vi "MS Operation IOP Ctrl.vi"(6 "PID Cluster":T3={"L1 to L4 PID Cluster"={"L1 PID Gains"={"Kp"=0.005, "Kd"=0.5, "Ki"=0.0005}, "L2 PID Gains"={"Kp"=0.01, "Kd"=1.0, "Ki"=0.005}, "L3 PID Gains"={"Kp"=0.05, "Kd"=1.0, "Ki"=0.0005}, "L4 PID Gains"={"Kp"=0.1, "Kd"=0.1, "Ki"=0.0005}}, "Stage PID Cluster"={"Stage Z PID"={"Kp"=0.0005, "Kd"=0.001, "Ki"=0.0}, "Stage Y PID"={"Kp"=0.0003, "Kd"=0.01, "Ki"=0.0}, "Stage X PID"={"Kp"=0.0003, "Kd"=0.01, "Ki"=0.0}}, "OCT Z PID Gains"={"Kp"=0.0003, "Kd"=0.0001, "Ki"=0.01}}, 8 "error in":errorcluster, 9 "Offset Home 2 RCM":dbl[](array[numeric])=[0.0, 0.0, 0.0, 0.0], 10 "Prev Posit Cluster":T2={"Prev L1 to L4 Posit"=[-0.5319, -0.035669172703475985, -2.0566170657346783, 0.9099264705882353], "Prev Stage Posit"=[6.002553885707208, 5.996566124542428, 5.995469940427586], "Prev OCT Z Posit"=-0.0}, 11 "FPGA VI Reference In":refnum<k20>) -> (0 "error out":errorcluster, 2 "Last Posit Cluster":T1={"Last L1 to L4 Posit"=[0.0, 0.0, 0.0, 0.0], "Last Stage Posit"=[6.0, 6.0, 6.0], "Last OCT Z Posit"=0.0}, 3 "FPGA VI Reference Out":refnum<k20>)   [LabVIEW 2016]
uses:
  Global Variables.vi
  <vilib>/Platform/TimedLoop/XDataNode/wakeup.ctl
  <vilib>/Platform/TimedLoop/XDataNode/XDNodeRunTimeDep.lvlib
  <vilib>/Platform/TimedLoop/XDataNode/nitl_modes.ctl
  <vilib>/Platform/TimedLoop/XDataNode/timing_clust.ctl
  <vilib>/platform/TimedLoop/XDataNode/XDataNode.xnode
  <vilib>/rvi/interface/nirviReadWriteControl/nirviReadWriteControl.xnode
  Library/KevinLibraryAll/labview/KevLib01.lvlib
  FPGA Bitfiles/PhantomControlPI_FPGATarget_QuadCtr2_E2412E44.lvbitx
  IRISS_FPGA_IO.vi
  <vilib>/Utility/error.llb/Error Cluster From Error Code.vi
  <vilib>/rvi/errors/niLvFpgaAdjustHostInterfaceError.vi
  <vilib>/Utility/file.llb/Write Delimited Spreadsheet (DBL).vi
  <vilib>/Utility/file.llb/Write Delimited Spreadsheet (string).vi
  NiFpgaLv.dll
panel:
  out "Period [ms]":i64=10
  out "Acc Button 4":bool
  out "Accurus Remote cmd":T4
  out "L1 to L4 Remote cmd":sgl[](array[numeric])
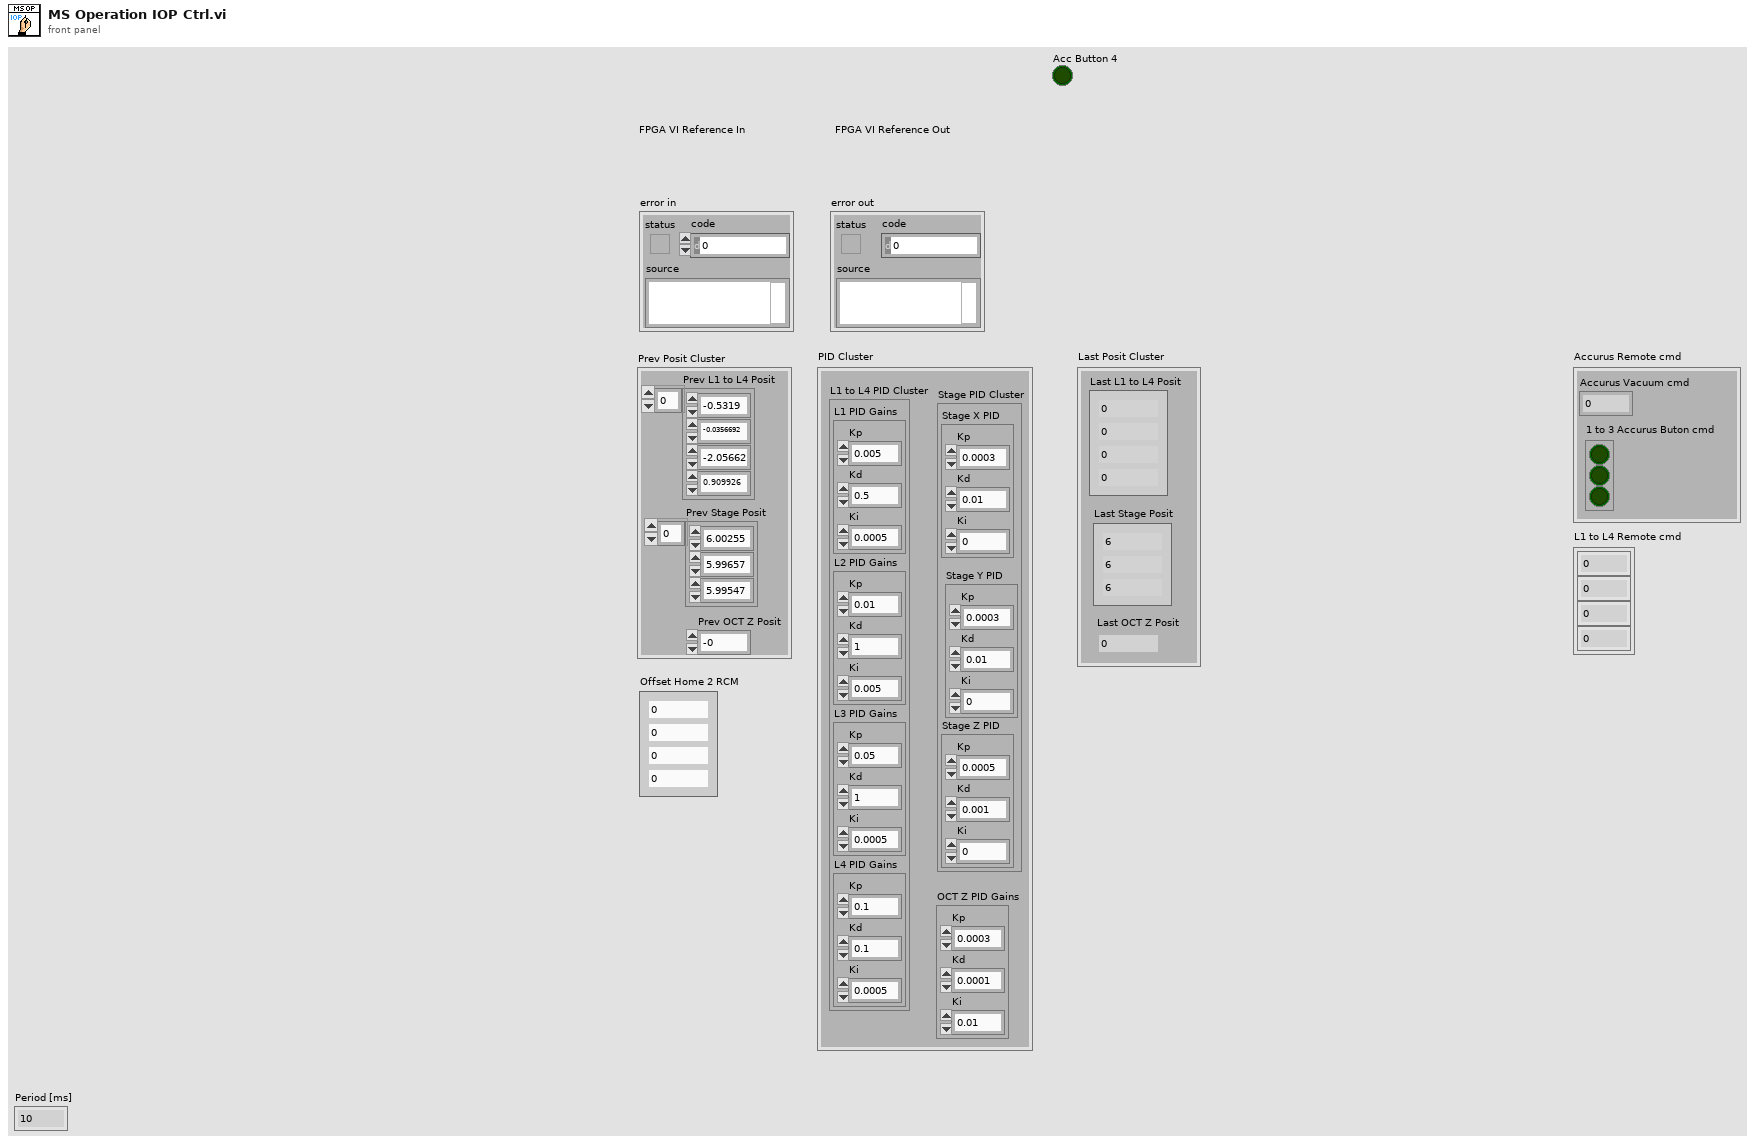
[diagram p1: front panel]
types:
  T1 = cluster{"Last L1 to L4 Posit":dbl[], "Last Stage Posit":dbl[], "Last OCT Z Posit":dbl}
  T2 = cluster{"Prev L1 to L4 Posit":dbl[], "Prev Stage Posit":dbl[], "Prev OCT Z Posit":dbl}
  T3 = cluster{"L1 to L4 PID Cluster":cluster{"L1 PID Gains":cluster{"Kp":dbl, "Kd":dbl, "Ki":dbl}, "L2 PID Gains":cluster{"Kp":dbl, "Kd":dbl, "Ki":dbl}, "L3 PID Gains":cluster{"Kp":dbl, "Kd":dbl, "Ki":dbl}, "L4 PID Gains":cluster{"Kp":dbl, "Kd":dbl, "Ki":dbl}}, "Stage PID Cluster":cluster{"Stage Z PID":cluster{"Kp":dbl, "Kd":dbl, "Ki":dbl}, "Stage Y PID":cluster{"Kp":dbl, "Kd":dbl, "Ki":dbl}, "Stage X PID":cluster{"Kp":dbl, "Kd":dbl, "Ki":dbl}}, "OCT Z PID Gains":cluster{"Kp":dbl, "Kd":dbl, "Ki":dbl}}
  T4 = cluster{"Accurus Vacuum cmd":sgl, "1 to 3 Accurus Buton cmd":bool[]}
  T5 = typedef "XDNodeRunTimeDep.lvlib/timing_clust.ctl" = cluster{"Expected End [f-1]":u64, "Actual End [f-1]":u64, "Finished Late? [f-1]":bool, "Expected End [i-1]":u64, "Actual End [i-1]":u64, "Finished Late? [i-1]":bool, "Expected Start [i]":u64, "Actual Start [i]":u64, "Expected Start [f]":u64, "Actual Start [f]":u64, "Source Name":string, "Structure Name":string, "Period":i64, "Deadline":i64, "Offset":i64, "Start":i64, "Priority":i32, "Timeout":i32, "Mode":T6, "Wakeup Reason":T7, "Error":errorcluster, "Source Type":string, "Secondary Source Type":string, "Global End Time":u64, "Global Start Time":u64, "Frame Duration":u64, "Iteration Duration":u64, "Assigned CPU":i32, "I/O Scan Engine Mode":u32}
  T6 = typedef "XDNodeRunTimeDep.lvlib/nitl_modes.ctl" = enum32{"No Change", "Process missed periods, maintain original phase", "Discard missed periods, maintain original phase", "Process missed periods, ignore original phase", "Discard missed periods, ignore original phase"}
  T7 = typedef "XDNodeRunTimeDep.lvlib/wakeup.ctl" = enum32{"Normal", "Aborted", "Asynchronous wakeup", "Timing source error", "Timed loop error", "Timeout"}
  T8 = cluster{"L1 PID Gains":cluster{"Kp":dbl, "Kd":dbl, "Ki":dbl}, "L2 PID Gains":cluster{"Kp":dbl, "Kd":dbl, "Ki":dbl}, "L3 PID Gains":cluster{"Kp":dbl, "Kd":dbl, "Ki":dbl}, "L4 PID Gains":cluster{"Kp":dbl, "Kd":dbl, "Ki":dbl}}
  T9 = cluster{"Stage Z PID":cluster{"Kp":dbl, "Kd":dbl, "Ki":dbl}, "Stage Y PID":cluster{"Kp":dbl, "Kd":dbl, "Ki":dbl}, "Stage X PID":cluster{"Kp":dbl, "Kd":dbl, "Ki":dbl}}
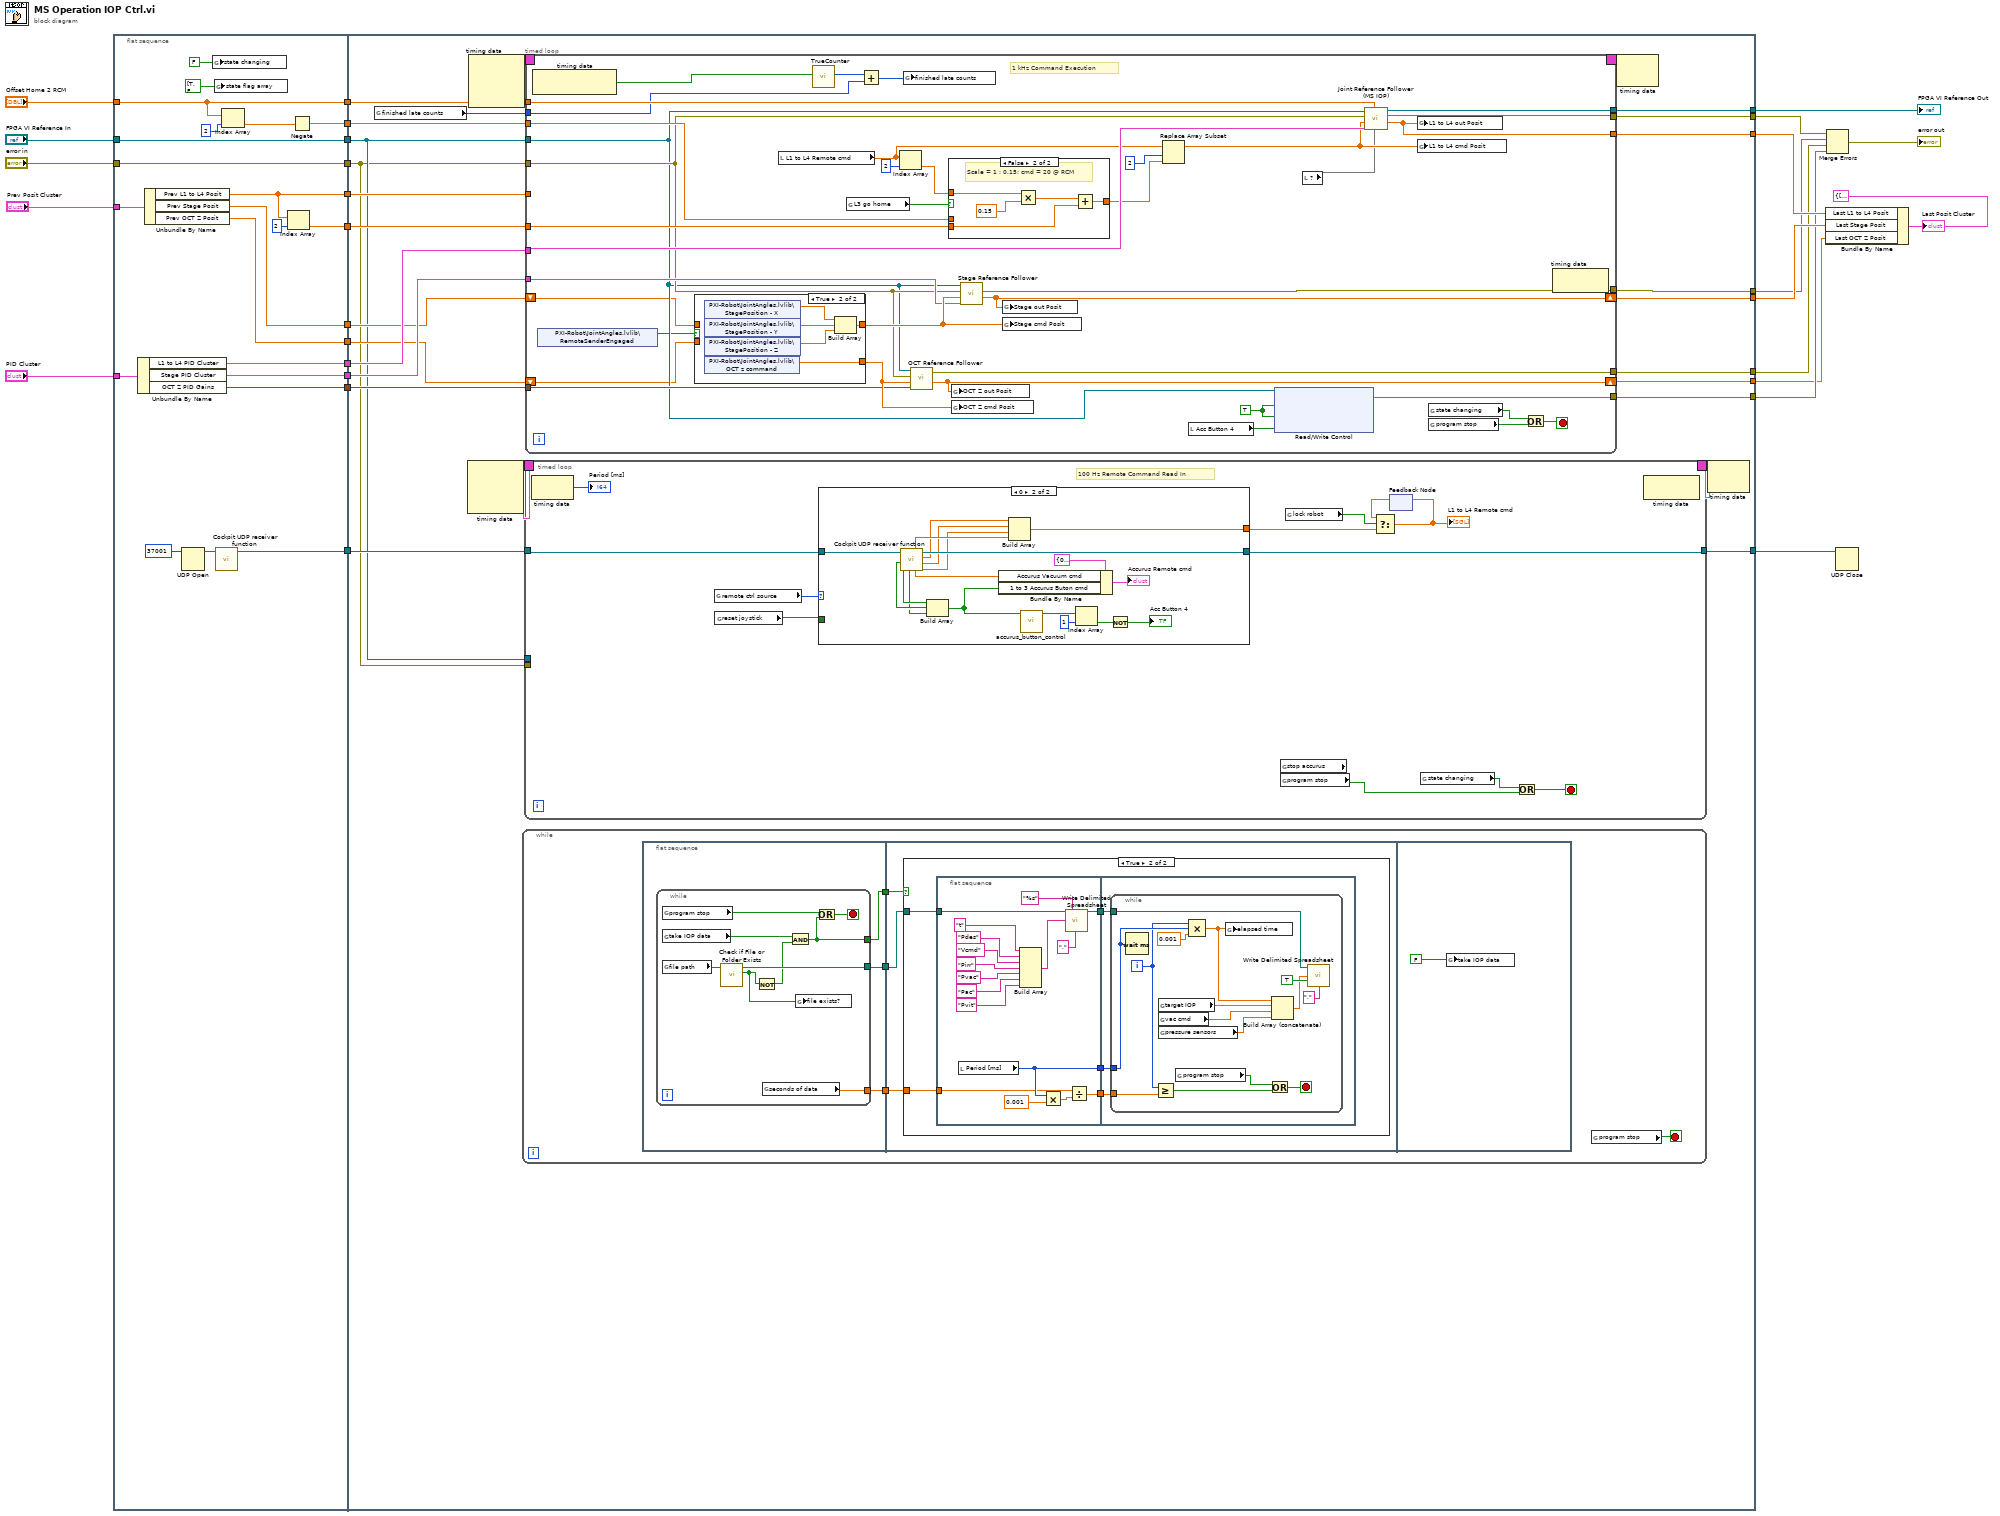
[diagram p0: block diagram]
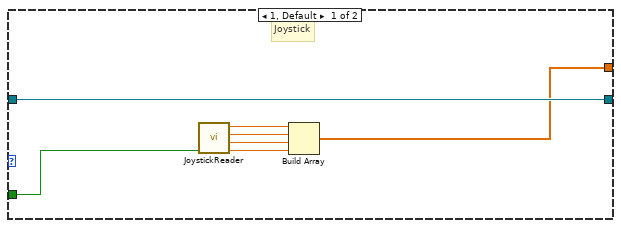
[diagram p3: hidden frame]
diagram:
  n1 = flat-sequence {
    tunnel: [w46] -> w29
    tunnel: [w45] -> w27
    tunnel: "FPGA VI Reference In" -> [w45]
    tunnel: [w44] -> w25
    tunnel: "error in" -> [w44]
    tunnel: [w37] -> w23
    tunnel: "Offset Home 2 RCM" -> [w37]
    tunnel: "Prev Posit Cluster" -> [w32]
    tunnel: [w42] -> w20
    tunnel: "PID Cluster" -> [w41]
    tunnel: [w40] -> w18
    tunnel: [w39] -> w17
    tunnel: [w35] -> w16
    tunnel: [w34] -> w4
    tunnel: [w33] -> w3
    tunnel: [w31] -> w2
    tunnel: [w30] -> w1
    tunnel: w29 -> [w72]
    tunnel: [w71] -> w28
    tunnel: w27 -> [w52]
    tunnel: w25 -> [w51]
    tunnel: w23 -> [w70]
    tunnel: w20 -> [w69]
    tunnel: w18 -> [w68]
    tunnel: w17 -> [w67]
    tunnel: w16 -> [w66]
    tunnel: [w65] -> w6
    tunnel: [w64] -> w12
    tunnel: [w63] -> w13
    tunnel: [w53] -> w10
    tunnel: [w54] -> w9
    tunnel: [w62] -> w7
    tunnel: [w61] -> w8
    tunnel: [w55] -> w5
    tunnel: w4 -> [w60]
    tunnel: w3 -> [w59]
    tunnel: w2 -> [w57]
    tunnel: w1 -> [w56]
    frame #0 {
      n2 = Unbundle By Name(w41) -> ("L1 to L4 PID Cluster"=w40:T8, "Stage PID Cluster"=w34:T9, "OCT Z PID Gains"=w33:cluster{"Kp":dbl, "Kd":dbl, "Ki":dbl})
      n3 = Unbundle By Name(w32) -> ("Prev L1 to L4 Posit"=w42:dbl[], "Prev Stage Posit"=w31:dbl[], "Prev OCT Z Posit"=w30:dbl)
      n4 = UDP Open(11:u16 37001 ("port")) -> (port=w48:refnum<k16>)  [unwired: 4 in, 2 out]
      n5 = global write "Global Variables.vi" "state changing"(FALSE ("state changing")) -> ()
      n6 = global write "Global Variables.vi" "state flag array"(bool[] [TRUE, FALSE, FALSE, FALSE, FALSE, FALSE, FALSE, FALSE, FALSE] ("state flag array")) -> ()
      n7 = call "Cockpit UDP receiver function.vi"("UDP connection ID"=w48) -> ("UDP connection ID out"=w46:refnum<k16>)  [unwired: 1 in, 9 out]
      n8 = Index Array(array=w37, index=2) -> (element=w36:dbl)
      n9 = Index Array(array=w42, index=2) -> (element=w39:dbl)
      n10 = Negate(x=w36) -> (-x=w35:dbl)
    }
    frame #1 {
      n11 = global read "Global Variables.vi" "finished late counts"() -> (w58:u16)
      n12 = node-c288() -> (w74:T5)  [unwired: 3 in]
      n13 = node-c288() -> (w76:T5)  [unwired: 3 in]
      n14 = while {
        stop <- w77 stop-if-true
        n15 = flat-sequence {
          tunnel: [w81] -> w80
          tunnel: [w83] -> w79
          tunnel: [w82] -> w78
          tunnel: w80 -> [w95]
          tunnel: w79 -> [w94]
          tunnel: w78 -> [w93]
          frame #0 {
            n16 = while {
              tunnel: [w91] -> w83
              tunnel: [w84] -> w82
              tunnel: [w89] -> w81
              stop <- w92 stop-if-true
              n17 = global read "Global Variables.vi" "program stop"() -> (w88:bool)
              n18 = global read "Global Variables.vi" "take IOP data"() -> (w87:bool)
              n19 = global read "Global Variables.vi" "file path"() -> (w86:path)
              n20 = call <vilib>:"Check if File or Folder Exists.vi"("path"=w86) -> ("file or folder exists?"=w85:bool, "dup path"=w91:path)  [unwired: 8 in, 1 out]
              n21 = Not(x=w85) -> (.not. x?=w90:bool)
              n22 = global read "Global Variables.vi" "seconds of data"() -> (w84:sgl)
              n23 = And(x=w87, y=w90) -> (x .and. y?=w89:bool)
              n24 = global write "Global Variables.vi" "file exists?"(w85) -> ()
              n25 = Or(x=w88, y=w89) -> (x .or. y?=w92:bool)
            }
          }
          frame #1 {
            n26 = case shown="True" w95 {
              tunnel: w94 -> [_ w100]
              tunnel: w93 -> [_ w97]
              frame False {
              }
              frame True {
                n27 = flat-sequence {
                  tunnel: w100 -> [w106]
                  tunnel: [w104] -> w99
                  tunnel: [w115] -> w98
                  tunnel: w97 -> [w114]
                  tunnel: [w112] -> w96
                  tunnel: w99 -> [w120]
                  tunnel: w98 -> [w119]
                  tunnel: w96 -> [w118]
                  frame #0 {
                    n28 = local read "Period [ms]"() -> (w115:i64)
                    n29 = Build Array("t" ("delimiter (\\t)"), "Pdes" ("delimiter (\\t)"), "Vcmd" ("delimiter (\\t)"), "Pirr" ("delimiter (\\t)"), "Pvac" ("delimiter (\\t)"), "Pac" ("delimiter (\\t)"), "Pvit" ("delimiter (\\t)")) -> (w103:string[])
                    n30 = Multiply(x=w115, y=0.001) -> (x*y=w113:dbl)
                    n31 = call-poly <vilib>:"Write Delimited Spreadsheet.vi"("file path (dialog if empty)"=w106, "format (%s)"="%s", "1D data"=w103, "delimiter (\\t)"="," ("delimiter (\\t)")) -> ("new file path (Not A Path if cancelled)"=w104:path)  [unwired: 10 in, 1 out]
                    n32 = Divide(x=w114, y=w113) -> (x/y=w112:dbl)
                  }
                  frame #1 {
                    n33 = while {
                      tunnel: w120 -> [w129]
                      tunnel: w119 -> [w133]
                      tunnel: w118 -> [w131]
                      i -> [w132]
                      stop <- w135 stop-if-true
                      n34 = Wait (ms)(milliseconds to wait=w133) -> ()  [unwired: 1 out]
                      n35 = Greater Or Equal?(x=w132, y=w131) -> (x >= y?=w130:bool)
                      n36 = global read "Global Variables.vi" "target IOP"() -> (w121:sgl)
                      n37 = global read "Global Variables.vi" "vac cmd"() -> (w124:sgl)
                      n38 = global read "Global Variables.vi" "pressure sensors"() -> (w123:sgl[])
                      n39 = global read "Global Variables.vi" "program stop"() -> (w125:bool)
                      n40 = Compound Arithmetic op=MULTIPLY(w132, w133, 0.001 ("y")) -> (w122:dbl)
                      n41 = global write "Global Variables.vi" "elapsed time"(w122) -> ()
                      n42 = Or(x=w125, y=w130) -> (x .or. y?=w135:bool)
                      n43 = Build Array (concatenate)(w122, w121, w124, w123) -> (w127:dbl[])
                      n44 = call-poly <vilib>:"Write Delimited Spreadsheet.vi"("file path (dialog if empty)"=w129, "1D data"=w127, "append to file? (new file:F)"=TRUE, "delimiter (\\t)"="," ("delimiter (\\t)")) -> ()  [unwired: 10 in, 2 out]
                    }
                  }
                }
              }
            }
          }
          frame #2 {
            n45 = global write "Global Variables.vi" "take IOP data"(FALSE) -> ()
          }
        }
        n46 = global read "Global Variables.vi" "program stop"() -> (w77:bool)
      }
      n47 = timed-loop {
        timing: w74 -> [_]
        timing-out: [_] -> w73
        tunnel: w72 -> [w146]
        tunnel: [w145] -> w71
        tunnel: w52 -> [_]
        tunnel: w51 -> [_]
        stop <- w148 stop-if-true
        # "100 Hz Remote Command Read In"
        n48 = node-c288() -> (→"Period [ms]":i64)  [unwired: 1 in]
        n49 = global read "Global Variables.vi" "remote ctrl source"() -> (w144:u16)
        n50 = global read "Global Variables.vi" "reset joystick"() -> (w143:bool)
        n51 = case shown="0" w144 {
          tunnel: [w154 w173] -> w145
          tunnel: w146 -> [w154 w163]
          tunnel: w143 -> [w155 _]
          tunnel: [w149 w162] -> w139
          frame 1, Default {
            # "Joystick"
            n52 = call "JoystickReader.vi"("Reset"=w155) -> ("L4 [deg]"=w150:sgl, "L3 [0~100]"=w151:sgl, "L2 [deg]"=w152:sgl, "L1 [deg]"=w153:sgl)  [unwired: 7 in]
            n53 = Build Array(w153, w152, w151, w150) -> (w149:sgl[])
          }
          frame 0 {
            n54 = call "Cockpit UDP receiver function.vi"("UDP connection ID"=w163) -> ("L3"=w170:sgl, "L2"=w169:sgl, "L1"=w171:sgl, "UDP connection ID out"=w173:refnum<k16>, "down_pedal"=w161:sgl, "L4"=w172:sgl, "right_pedal"=w164:bool, "left_pedal"=w166:bool, "up_pedal"=w165:bool)  [unwired: 1 in, 1 out]
            n55 = Build Array(w166, w165, w164) -> (w156:bool[])
            n56 = Bundle By Name(cluster=T4 {"Accurus Vacuum cmd"=0.0, "1 to 3 Accurus Buton cmd"=[FALSE, FALSE, FALSE]} ("Accurus Cockpit cmd 2"), "Accurus Vacuum cmd"=w161, "1 to 3 Accurus Buton cmd"=w156) -> (→"Accurus Remote cmd":T4)
            n57 = Build Array(w171, w169, w170, w172) -> (w162:sgl[])
            n58 = call "accurus_button_control.vi"("Array in"=w156) -> ("Array out"=w159:bool[])  [unwired: 10 in]
            n59 = Index Array(array=w159, index=1) -> (element=w158:bool)
            n60 = Not(x=w158) -> (.not. x?=→"Acc Button 4":bool)
          }
        }
        n61 = global read "Global Variables.vi" "stop accurus"() -> ()  [unwired: 1 out]
        n62 = global read "Global Variables.vi" "program stop"() -> (w138:bool)
        n63 = global read "Global Variables.vi" "lock robot"() -> (w142:bool)
        n64 = feedback #1() -> (w141:sgl[])  [unwired: 1 in]
        n65 = Select(t=w141, s=w142, f=w139) -> (s? t:f=w140:sgl[])
        "L1 to L4 Remote cmd" <- w140
        n66 = feedback-in #1(w140) -> ()
        n67 = global read "Global Variables.vi" "state changing"() -> (w147:bool)
        n68 = Or(x=w147, y=w138) -> (x .or. y?=w148:bool)
        n69 = node-c288() -> ()  [unwired: 1 in, 1 out]
      }
      n70 = timed-loop {
        timing: w76 -> [_]
        timing-out: [_] -> w75
        tunnel: w52 -> [w189]
        tunnel: w51 -> [w190]
        tunnel: w70 -> [w211]
        tunnel: w69 -> [_]
        tunnel: w68 -> [w208]
        tunnel: w67 -> [w207]
        tunnel: w66 -> [w204]
        tunnel: [w203] -> w65
        tunnel: [w202] -> w64
        tunnel: [w201] -> w63
        tunnel: [w200] -> w62
        tunnel: [w199] -> w61
        tunnel: w60 -> [w196]
        tunnel: w59 -> [w195]
        tunnel: w58 -> [w191]
        shift-right: [w185] -> w54
        shift-left: w57 -> [w188]
        shift-right: [w186] -> w55
        shift-left: w56 -> [w187]
        tunnel: [w182] -> w53
        stop <- w216 stop-if-true
        w198 = TRUE ("Conn0/DIO15 Button 4")
        # "1 kHz Command Execution"
        n71 = node-c288() -> (w194:bool)  [unwired: 1 in]
        n72 = shared-variable "PXI-Robot\\JointAngles.lvlib\\RemoteSenderEngaged"() -> (w184:bool)  [unwired: 1 in, 1 out]
        n73 = case shown="True" w184 {
          tunnel: [w218 w223] -> w210
          tunnel: [w217 w219] -> w209
          tunnel: w188 -> [w218 _]
          tunnel: w187 -> [w217 _]
          frame False {
          }
          frame True {
            n74 = shared-variable "PXI-Robot\\JointAngles.lvlib\\StagePosition - X"() -> (w220:dbl)  [unwired: 1 in, 1 out]
            n75 = shared-variable "PXI-Robot\\JointAngles.lvlib\\StagePosition - Y"() -> (w221:dbl)  [unwired: 1 in, 1 out]
            n76 = shared-variable "PXI-Robot\\JointAngles.lvlib\\StagePosition - Z"() -> (w222:dbl)  [unwired: 1 in, 1 out]
            n77 = shared-variable "PXI-Robot\\JointAngles.lvlib\\OCT z command"() -> (w219:dbl)  [unwired: 1 in, 1 out]
            n78 = Build Array(w220, w221, w222) -> (w223:dbl[])
          }
        }
        n79 = local read "L1 to L4 Remote cmd"() -> (w183:sgl[])
        n80 = call "TrueCounter.vi"("True?"=w194) -> ("True Count"=w192:u16)  [unwired: 10 in]
        n81 = global read "Global Variables.vi" "L3 go home"() -> (w214:bool)
        n82 = Add(x=w192, y=w191) -> (x+y=w193:u16)
        n83 = Index Array(array=w183, index=2) -> (element=w212:sgl)
        n84 = global write "Global Variables.vi" "finished late counts"(w193) -> ()
        n85 = call "OCT Reference Follower.vi"("OCT Z PID Gains"=w195, "OCT  Z cmd Posit [mm]"=w209, "error in"=w190, "FPGA VI Reference In"=w189) -> ("OCT  Z out Posit [mm]"=w186:dbl, "error out"=w200:errorcluster)  [unwired: 5 in, 1 out]
        n86 = case shown="False" w214 {
          tunnel: [w224 w229] -> w205
          tunnel: w212 -> [_ w226]
          tunnel: w207 -> [_ w225]
          tunnel: w204 -> [w224 _]
          frame True {
            # "Go Home"
          }
          frame False {
            # "Scale = 1 : 0.15; cmd = 20 @ RCM"
            n87 = Multiply(x=w226, y=0.15) -> (x*y=w228:dbl)
            n88 = Add(x=w228, y=w225) -> (x+y=w229:dbl)
          }
        }
        n89 = global write "Global Variables.vi" "OCT Z out Posit"(w186) -> ()
        n90 = global write "Global Variables.vi" "OCT Z cmd Posit"(w209) -> ()
        n91 = call "Stage Reference Follower.vi"("Stage PID Cluster"=w196, "Stage cmd Posit [mm]"=w210, "error in"=w190, "FPGA VI Reference In"=w189) -> ("Stage out Posit [mm]"=w185:dbl[], "error out"=w199:errorcluster)  [unwired: 5 in, 1 out]
        n92 = global write "Global Variables.vi" "Stage out Posit"(w185) -> ()
        n93 = global write "Global Variables.vi" "Stage cmd Posit"(w210) -> ()
        n94 = Replace Array Subset(array=w183, new element=w205, index=2) -> (w181:sgl[])
        n95 = local read "Acc Button 4"() -> (w179:bool)
        n96 = xnode "Read/Write Control"("FPGA VI Reference In"=w189, "Conn0/DIO12 Button 1"=w198, "Conn0/DIO13 Button 2"=w198, "Conn0/DIO15 Button 4"=w179) -> ("error out"=w203:errorcluster)  [unwired: 1 in, 1 out]
        n97 = local read item#-1() -> (w180)
        n98 = call "Joint Reference Follower (MS IOP).vi"("Acc Ctrl Array"=w180, "Offset Home2RCM [deg/mm]"=w211, "PID Ctrl Cluster"=w208, "Ref Array [deg/mm]"=w181, "error in"=w190, "FPGA VI Reference In"=w189) -> ("Output Posit Array [deg/mm]"=w182:dbl[], "error out"=w202:errorcluster, "FPGA VI Reference Out"=w201:refnum<k20>)  [unwired: 3 in]
        n99 = global write "Global Variables.vi" "L1 to L4 out Posit"(w182) -> ()
        n100 = global write "Global Variables.vi" "L1 to L4 cmd Posit"(w181) -> ()
        n101 = global read "Global Variables.vi" "state changing"() -> (w215:bool)
        n102 = global read "Global Variables.vi" "program stop"() -> (w197:bool)
        n103 = Or(x=w215, y=w197) -> (x .or. y?=w216:bool)
        n104 = node-c288() -> ()  [unwired: 1 in, 1 out]
      }
      n105 = node-c288(w75) -> ()  [unwired: 1 out]
      n106 = node-c288(w73) -> ()  [unwired: 1 out]
    }
  }
  n107 = Bundle By Name(cluster=T1 {"Last L1 to L4 Posit"=[-0.5607, -0.038216970753724266, -2.0806193533568895, 1.1787683823529411], "Last Stage Posit"=[6.002553885707208, 5.996566124542428, 5.995469940427586], "Last OCT Z Posit"=-0.0} ("Last Posit Cluster 2"), "Last L1 to L4 Posit"=w10, "Last Stage Posit"=w9, "Last OCT Z Posit"=w5) -> (→"Last Posit Cluster":T1)
  n108 = Merge Errors(w12, w8, w7, w6) -> (→"error out":errorcluster)
  n109 = UDP Close(connection ID=w28) -> ()  [unwired: 1 in, 2 out]
  "FPGA VI Reference Out" <- w13
